vi "Passwort.vi"(0 "Enable":bool=TRUE caption="Aktivieren", 5 "error in (no error)":errorcluster caption="Fehler (Eingang, kein Fehler)") -> (17 "Passwort":string, 18 "OK":bool, 19 "error out":errorcluster caption="Fehler (Ausgang)")   [LabVIEW 2010]
doc: "Zeigt ein Standarddialogfeld an, das den Anwender zur Eingabe von Informationen (zum Beispiel von Name und Passwort) auffordert.\n--------------------\n\nDieses Express-VI ist wie folgt konfiguriert:\n\nMeldung zur Ausgabe an den Benutzer:Bitte Passwort eingeben\nDie Eingaben sind: \nZahlenwert: Passwort"
panel:
  in  "Passwort":string
  in  "Passwort:":string caption="Passwort"
  out "String":string="Bitte Passwort eingeben"
  in  "Cancel":bool caption="Abbrechen"
  in  "OK2":bool
  in  "OK1":bool
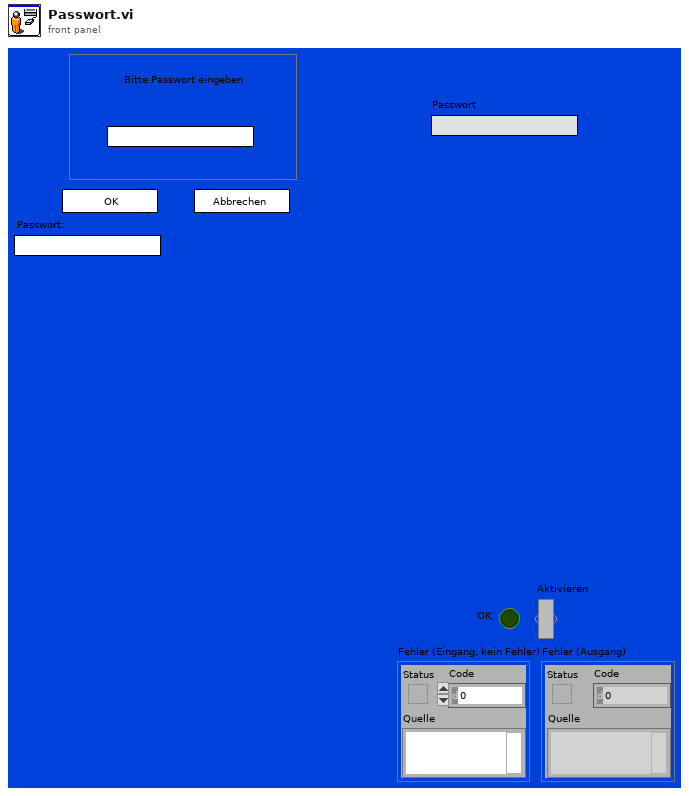
[diagram p1: front panel]
types:
  T1 = cluster{"Input Name":string, "Input Data Type":i32}[]
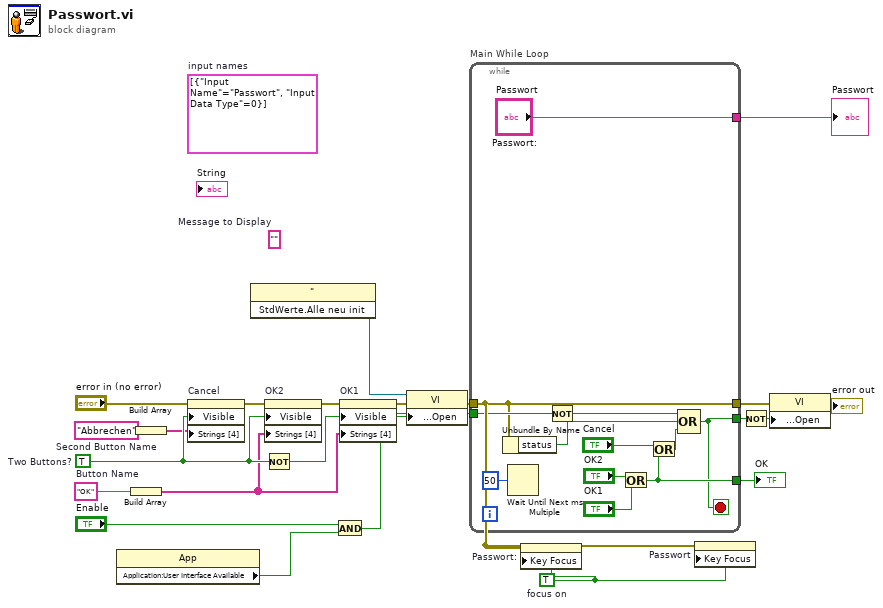
[diagram p0: block diagram]
diagram:
  w1 = TRUE  # focus on
  (unwired) T1 [{"Input Name"="Passwort", "Input Data Type"=0}]  # input names
  w14 = "Abbrechen"  # Second Button Name
  w12 = "OK"  # Button Name
  (unwired) ""  # Message to Display
  w22 = TRUE  # Two Buttons?
  n1 = property class="App"() -> ("Application:User Interface Available"=w4:bool)  [unwired: 2 in, 2 out]
  n2 = Build Array(w12) -> (w13:string[])
  n3 = Build Array(w14) -> (w15:string[])
  n4 = property on="Cancel" class="Bool."(error in="error in (no error)", "Visible"=w22, "Strings [4]"=w15) -> (error out=w19:errorcluster)  [unwired: 1 in, 1 out]
  n5 = invoke class="\"" method="StdWerte.Alle neu init"() -> (reference out=w3:refnum<vi>)  [unwired: 3 in, 2 out]
  n6 = Not(x=w22) -> (.not. x?=w20:bool)
  n7 = property on="OK2" class="Bool."(error in=w19, "Visible"=w22, "Strings [4]"=w13) -> (error out=w18:errorcluster)  [unwired: 1 in, 1 out]
  n8 = And(x="Enable", y=w4) -> (x .and. y?=w5:bool)
  n9 = property on="OK1" class="Bool."(error in=w18, "Visible"=w20, "Strings [4]"=w13) -> (error out=w11:errorcluster)  [unwired: 1 in, 1 out]
  n10 = property class="VI"(reference=w3, error in=w11, "Front Panel Window:Open"=w5) -> (error out=w10:errorcluster)  [unwired: 1 out]
  n11 = while "Main While Loop" {
    tunnel: [w32] -> w21
    tunnel: w5 -> [w30]
    tunnel: [w28] -> w16
    tunnel: w10 -> [w27]
    tunnel: [w27] -> w8
    tunnel: ["Passwort:"] -> _
    tunnel: ["Passwort"] -> w2
    stop <- w28 stop-if-true
    n12 = Unbundle By Name(w27) -> ("status"=w25:bool)
    n13 = Wait Until Next ms Multiple(millisecond multiple=u32 50) -> ()  [unwired: 1 out]
    n14 = Not(x=w30) -> (.not. x?=w29:bool)
    n15 = Or(x="OK2", y="OK1") -> (x .or. y?=w32:bool)
    n16 = Or(x="Cancel", y=w32) -> (x .or. y?=w26:bool)
    n17 = Compound Arithmetic op=OR(w29, w25, w26) -> (w28:bool)
  }
  "OK" <- w21
  "Passwort" <- w2
  n18 = property on="Passwort:" class="Str"(error in=w10, "Key Focus"=w1) -> ()  [unwired: 1 in, 2 out]
  n19 = property on="Passwort" class="Str"(error in=w10, "Key Focus"=w1) -> ()  [unwired: 1 in, 2 out]
  n20 = Not(x=w16) -> (.not. x?=w17:bool)
  n21 = property class="VI"(error in=w8, "Front Panel Window:Open"=w17) -> (error out=→"error out":errorcluster)  [unwired: 1 in, 1 out]
